vi "Destroy.vi"(0 "reference in":refnum<class "VINode.lvclass">, 5 "error in (no error)":errorcluster) -> (14 "reference out":refnum<class "VINode.lvclass">, 19 "error out":errorcluster)   [LabVIEW 2016, in "VINode.lvclass"]
doc: "Destroys a ClassNode object created with a ClassNode constructor VI.\n\n[GOOP 2.1]"
uses:
  <resource>/Framework/Providers/Open_GDS/UML/VINode_class/VINode.lvclass
  <resource>/Framework/Providers/Open_GDS/UML/RectangularNode_class/RectangularNode.lvclass
  <resource>/Framework/Providers/Open_GDS/UML/MultiLineString_class/MultiLineString.lvclass
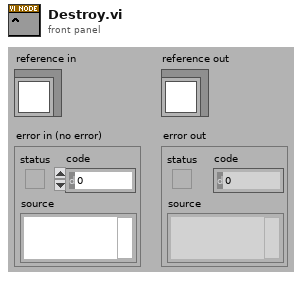
[diagram p1: front panel]
types:
  T1 = typedef "VINode.lvclass/ObjectAttributes.ctl" = cluster{"midHeight":dbl, "botHeight":dbl, "Name":refnum<class "MultiLineString.lvclass">, "DEFAULT_COMPARTMENT_HEIGHT":i32, "DEFAULT_WIDTH":i32, "DEFAULT_HEIGHT":i32, "VIPath":path, "Description":refnum<class "MultiLineString.lvclass">, "ShowDescription":bool}
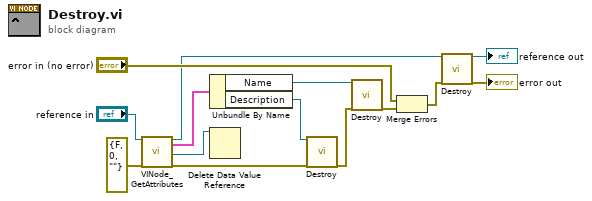
[diagram p0: block diagram]
diagram:
  n1 = call <resource>:"VINode_GetAttributes.vi"("reference in"="reference in", "error in (no error)"=errorcluster {"status"=FALSE, "code"=0, "source"=""}) -> ("reference out"=w5:refnum<class "VINode.lvclass">, "Data"=w7:T1, "DataRef"=w6:refnum<data-value>, "error out"=w2:errorcluster)  [unwired: 1 in, 13 out]
  n2 = Unbundle By Name(w7) -> ("Name"=w10:refnum<class "MultiLineString.lvclass">, "Description"=w3:refnum<class "MultiLineString.lvclass">)
  n3 = Delete Data Value Reference(data value reference=w6) -> ()  [unwired: 1 in, 2 out]
  n4 = call-dynamic "Destroy.vi"("reference"=w3, "error in (no error)"=w2) -> ("error out"=w1:errorcluster)  [unwired: 16 in, 1 out]
  n5 = call-dynamic "Destroy.vi"("reference"=w10, "error in (no error)"=w1) -> ("error out"=w9:errorcluster)  [unwired: 16 in, 1 out]
  n6 = Merge Errors("error in (no error)", w9) -> (w8:errorcluster)
  n7 = call-parent "Destroy.vi"("reference"=w5, "error in (no error)"=w8) -> ("reference out"=→"reference out":refnum<class "VINode.lvclass">, "error out"=→"error out":errorcluster)  [unwired: 16 in]
